vi "KVMap-AppendStrToKey.vi"(10 "string":string, 11 "Cluster in":cluster{string[], string[]}) -> (3 "Cluster out":cluster{string[], string[]})   [LabVIEW 2014]
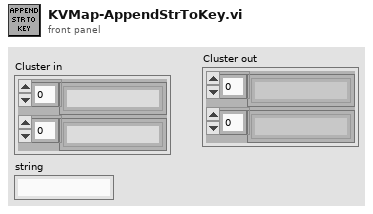
[diagram p1: front panel]
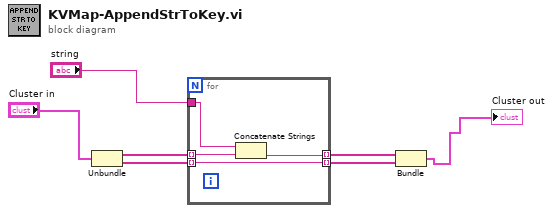
[diagram p0: block diagram]
diagram:
  n1 = Unbundle("Cluster in") -> (w2:string[], w7:string[])
  n2 = for {
    tunnel: w2 -> [w11] mode=indexing
    tunnel: w7 -> [w10] mode=indexing
    tunnel: [w10] -> w4 mode=indexing
    tunnel: [w9] -> w3 mode=indexing
    tunnel: "string" -> [w8]
    n3 = Concatenate Strings(w8, w11) -> (w9:string)
  }
  n4 = Bundle(w3, w4) -> (→"Cluster out":cluster{string[], string[]})  [unwired: 1 in]
